vi "Get Offset.vi"(8 "error in (no error)":errorcluster, 10 "Channel":T1, 11 "EPU452 in":refnum<class "EPU452.lvclass">) -> (0 "error out":errorcluster, 1 "Offset":dbl, 2 "Response":string, 3 "EPU452 out":refnum<class "EPU452.lvclass">)   [LabVIEW 2018, in "EPU452.lvclass"]
uses:
  EPU452.lvclass
  Controls/Channels.ctl
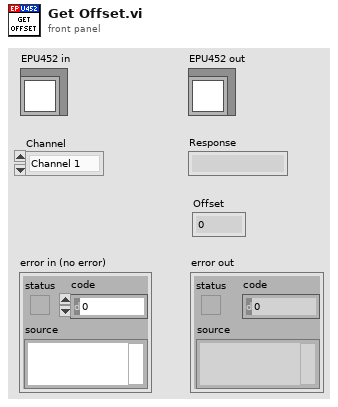
[diagram p1: front panel]
types:
  T1 = typedef "EPU452.lvclass/Channels.ctl" = enum16{"Channel 1", "Channel 2", "Channel 3", "Channel 4"}
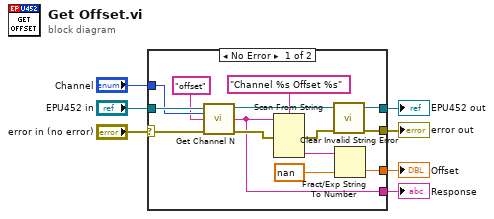
[diagram p0: block diagram]
diagram:
  n1 = case shown="No Error" "error in (no error)" {
    selector: "error in (no error)" -> [w19 w23]
    tunnel: [w12 w23] -> w6
    tunnel: [w11 w22] -> w4
    tunnel: "EPU452 in" -> [w21 w22]
    tunnel: "Channel" -> [w20 _]
    tunnel: [w10 _] -> w2
    tunnel: [w9 _] -> w1
    frame No Error {
      n2 = call "Get Channel N.vi"("EPU452 in"=w21, "Channel"=w20, "Function"="offset", "error in (no error)"=w19) -> ("EPU452 out"=w16:refnum<class "EPU452.lvclass">, "Response"=w9:string, "error out"=w17:errorcluster)  [unwired: 9 in]
      n3 = Scan From String(format string="Channel %s Offset %s", input string=w9, error in=w17) -> (error out=w14:errorcluster, output 2=w13:string)  [unwired: 4 in, 2 out]
      n4 = call "Clear Invalid String Error.vi"("error in (no error)"=w14, "EPU452 in"=w16) -> ("error out"=w12:errorcluster, "EPU452 out"=w11:refnum<class "EPU452.lvclass">)  [unwired: 8 in]
      n5 = Fract/Exp String To Number(string=w13, default (0 dbl)=nan ("default (0 DBL)")) -> (number=w10:dbl)  [unwired: 2 in, 1 out]
    }
    frame Error {
    }
  }
  "error out" <- w6
  "EPU452 out" <- w4
  "Offset" <- w2
  "Response" <- w1
